vi "HVOF_DAQ.vi"() -> ()   [LabVIEW 2018]
uses:
  <vilib>/Enthought/Python Integration Toolkit/api/Console Visibility.ctl
  Global Variables.vi
  <vilib>/Enthought/Python Integration Toolkit/api/Unpack Double Array.vi
  <resource>/objmgr/daqmx.rc
  <vilib>/Enthought/Python Integration Toolkit/Python Integration Toolkit.lvlib
panel:
  out "Delta T (water)":cluster{"X":dbl[], "Y":dbl[]}(graph)
  in  "Clear Graph":bool=TRUE
  out "XY Graph":cluster{"Y":dbl[], "Y":dbl[]}[](graph)
  in  "Enum":T1(ring)
  out "Data":T2 {"O2 Flow" scale=0.0..600.0; "Fuel Flow" scale=0.0..16.0}
  in  "Temperatures Task Name":refnum<k21>
  in  "Currents Task Name":refnum<k21>
  in  "stop":bool
  # "HVOF"
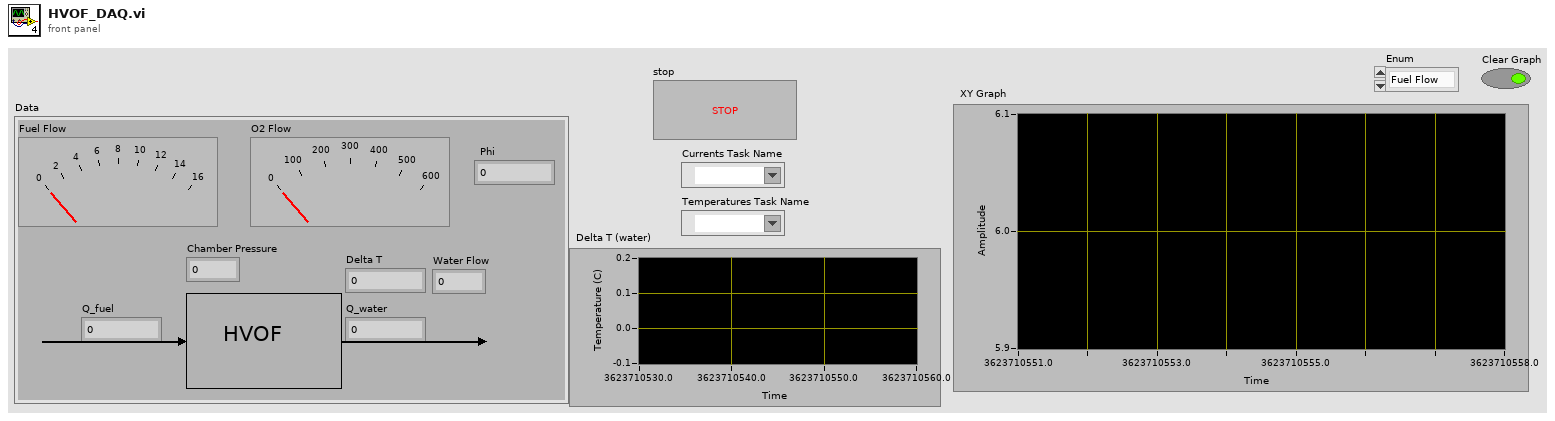
[diagram p1: front panel]
types:
  T1 = enum16{"Fuel Flow", "O2 Flow", "Phi", "Q_water", "Q_Fuel", "Delta T", "Water Flow", "Chamber Pressure"}
  T2 = cluster{"Fuel Flow":dbl, "O2 Flow":dbl, "Phi":dbl, "Q_water":dbl, "Q_fuel":dbl, "Delta T":dbl, "Water Flow":dbl, "Chamber Pressure":dbl}
  T3 = typedef "Python Integration Toolkit.lvlib/Console Visibility.ctl" = enum16{"Show Console", "Show Console While Running", "Hide Console"}
  T4 = typedef "Python Integration Toolkit.lvlib/Session ID.ctl" = u64
  T5 = typedef "Python Integration Toolkit.lvlib/Python Objects.ctl" = variant
  T6 = cluster{dbl, dbl, "Numeric":dbl, "Numeric":dbl, "Numeric":dbl, dbl, dbl, dbl}
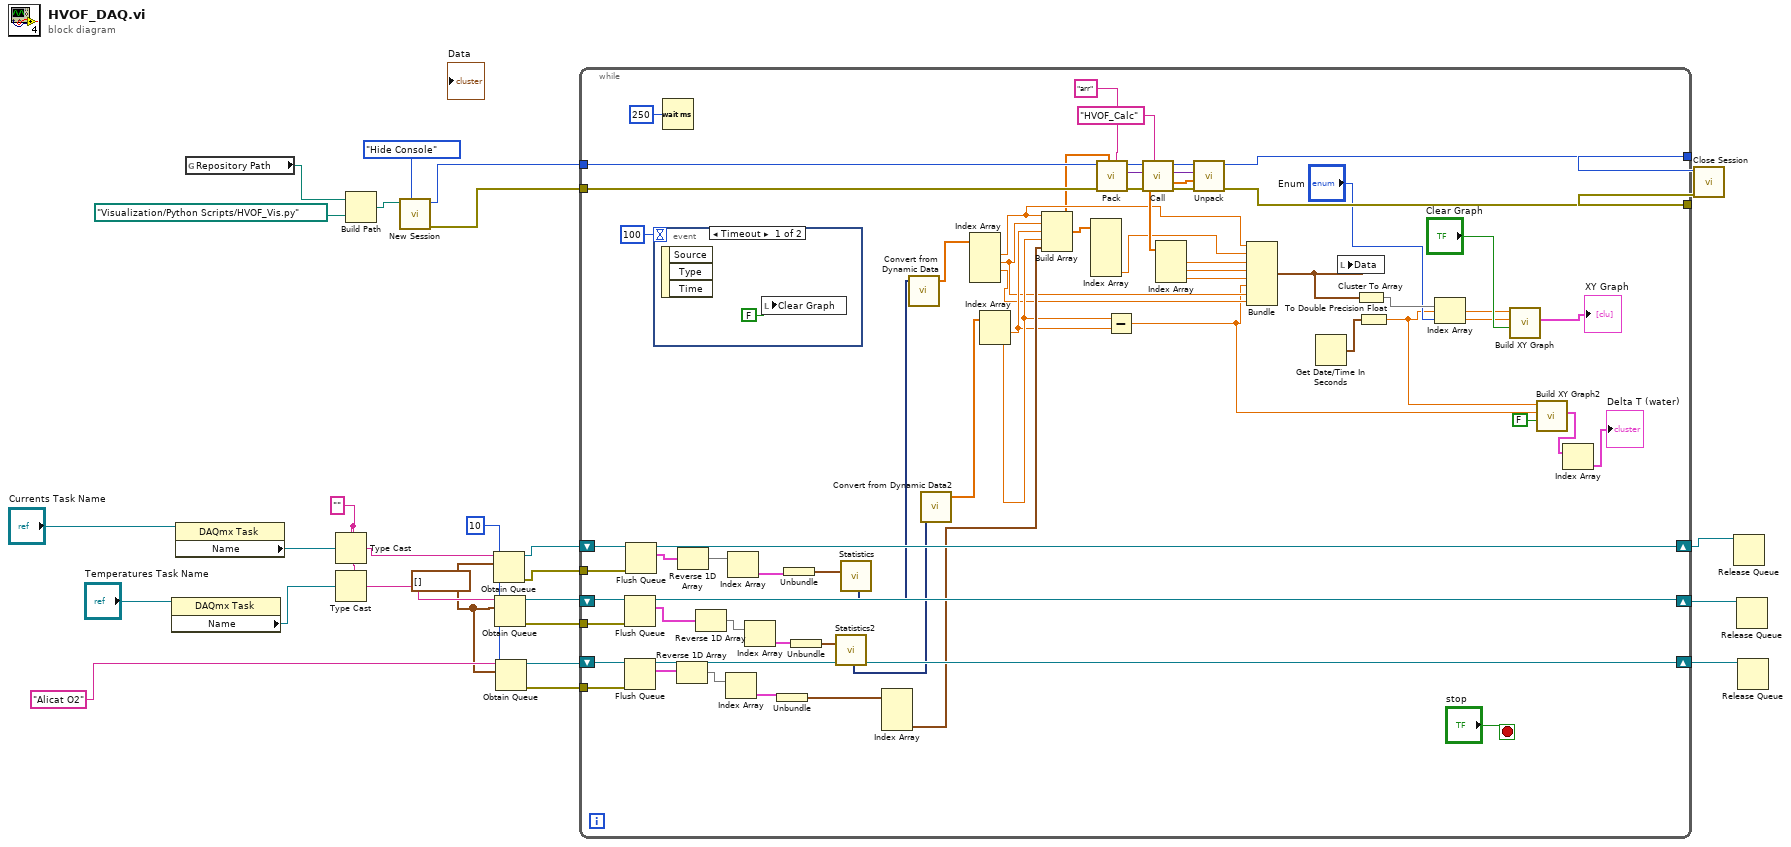
[diagram p0: block diagram]
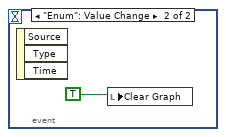
[diagram p2: hidden frame]
diagram:
  w15 = waveform(dbl)[] [] ("data")
  w4 = 10 ("max queue size (-1, unlimited)")
  w25 = "" ("type")
  n1 = property class="DAQmx Task"(reference="Temperatures Task Name") -> ("Name"=w23:refnum<k21>)  [unwired: 1 in, 2 out]
  n2 = property class="DAQmx Task"(reference="Currents Task Name") -> ("Name"=w27:refnum<k21>)  [unwired: 1 in, 2 out]
  n3 = global read "Global Variables.vi" "Repository Path"() -> (w9:path)
  n4 = Type Cast(type=w25, x=w27) -> (*(type *) &x=w26:string)
  n5 = Type Cast(type=w25, x=w23) -> (*(type *) &x=w24:string)
  n6 = Build Path(base path=w9, name or relative path=path "Visualization/Python Scripts/HVOF_Vis.py" ("vi path")) -> (appended path=w11:path)
  n7 = call <vilib>:"New Session.vi"("Console Visibility"=Console_Visibility."Hide Console", "Path to Python Module (.py File)"=w11) -> ("error out"=w7:errorcluster, "Session ID out"=w8:T4)  [unwired: 8 in]
  n8 = Obtain Queue(max queue size (-1, unlimited)=w4, name (unnamed)=w26, element data type=w15) -> (queue out=w20:refnum<queue>, error out=w18:errorcluster)  [unwired: 2 in, 1 out]
  n9 = Obtain Queue(max queue size (-1, unlimited)=w4, name (unnamed)=w24, element data type=w15) -> (queue out=w19:refnum<queue>, error out=w17:errorcluster)  [unwired: 2 in, 1 out]
  n10 = Obtain Queue(max queue size (-1, unlimited)=w4, name (unnamed)="Alicat O2", element data type=w15) -> (queue out=w14:refnum<queue>, error out=w13:errorcluster)  [unwired: 2 in, 1 out]
  n11 = while {
    shift-right: [w87] -> w2
    shift-left: w19 -> [w89]
    shift-right: [w88] -> w3
    shift-left: w20 -> [w90]
    tunnel: w18 -> [w84]
    tunnel: w17 -> [w83]
    shift-right: [w72] -> w1
    shift-left: w14 -> [w75]
    tunnel: w13 -> [w71]
    tunnel: w8 -> [w70]
    tunnel: w7 -> [w69]
    tunnel: [w60] -> w6
    tunnel: [w59] -> w5
    stop <- "stop" stop-if-true
    n12 = Flush Queue(queue=w89, error in (no error)=w83) -> (queue out=w87:refnum<queue>, remaining elements=w86:cluster{"data":waveform(dbl)[]}[])  [unwired: 1 out]
    n13 = Flush Queue(queue=w75, error in (no error)=w71) -> (queue out=w72:refnum<queue>, remaining elements=w73:cluster{"data":waveform(dbl)[]}[])  [unwired: 1 out]
    n14 = Flush Queue(queue=w90, error in (no error)=w84) -> (queue out=w88:refnum<queue>, remaining elements=w85:cluster{"data":waveform(dbl)[]}[])  [unwired: 1 out]
    n15 = event shown="[0] Timeout" {
      selector: _ -> [_ _]
      dyn-events: _ -> [_ _]
      timeout: 100 -> [_ _]
      event Timeout {
        n16 = event-data() -> ()  [unwired: 1 in, 3 out]
        n17 = local write "Clear Graph"(FALSE) -> ()
      }
      event "Enum": Value Change {
        n18 = event-data() -> ()  [unwired: 1 in, 3 out]
        n19 = local write "Clear Graph"(TRUE) -> ()
      }
    }
    n20 = Wait (ms)(milliseconds to wait=u32 250) -> ()  [unwired: 1 out]
    n21 = Reverse 1D Array(array=w73) -> (reversed array=w74:cluster{"data":waveform(dbl)[]}[])
    n22 = Reverse 1D Array(array=w85) -> (reversed array=w82:cluster{"data":waveform(dbl)[]}[])
    n23 = Reverse 1D Array(array=w86) -> (reversed array=w81:cluster{"data":waveform(dbl)[]}[])
    n24 = Index Array(array=w74) -> (element=w54:cluster{"data":waveform(dbl)[]})  [unwired: 1 in]
    n25 = Index Array(array=w82) -> (element=w80:cluster{"data":waveform(dbl)[]})  [unwired: 1 in]
    n26 = Index Array(array=w81) -> (element=w79:cluster{"data":waveform(dbl)[]})  [unwired: 1 in]
    n27 = Unbundle(w54) -> ("data"=w53:waveform(dbl)[])
    n28 = Unbundle(w80) -> ("data"=w77:waveform(dbl)[])
    n29 = Unbundle(w79) -> ("data"=w76:waveform(dbl)[])
    n30 = call "Statistics2"("Signals"=w76) -> ("Arithmetic Mean"=w57:dynamicdata)  [unwired: 25 in, 1 out]
    n31 = call "Statistics"("Signals"=w77) -> ("Arithmetic Mean"=w58:dynamicdata)  [unwired: 25 in, 1 out]
    n32 = Index Array(array=w53) -> (element #3=w47:waveform(dbl))  [unwired: 3 in, 2 out]
    n33 = call "Convert from Dynamic Data"("Dynamic Data Type"=w58) -> ("Array"=w56:dbl[])  [unwired: 3 in]
    n34 = call "Convert from Dynamic Data2"("Dynamic Data Type"=w57) -> ("Array"=w55:dbl[])  [unwired: 3 in]
    n35 = Index Array(array=w56) -> (element #1=w48:dbl, element #2=w35:dbl, element #3=w34:dbl)  [unwired: 4 in, 1 out]
    n36 = Index Array(array=w55) -> (element #1=w45:dbl, element #2=w46:dbl)  [unwired: 2 in]
    n37 = Build Array(w48, w35, w45, w46, w47) -> (w43:dbl[])
    n38 = Index Array(array=w43) -> (element #5=w42:dbl)  [unwired: 5 in, 4 out]
    n39 = call <vilib>:"Pack.vi"("Keyword Name"="arr", "Argument"=w43, "error in (no error)"=w69, "Session ID"=w70) -> ("error out"=w68:errorcluster, "Python Object References Out"=w67:T5, "Session ID out"=w66:T4)  [unwired: 5 in]
    n40 = Subtract(x=w46, y=w45) -> (x-y=w33:dbl)
    n41 = call <vilib>:"Call.vi"("Function or Method Name"="HVOF_Calc" ("Python Code"), "error in (no error)"=w68, "Python Object References In"=w67, "Session ID"=w66) -> ("error out"=w63:errorcluster, "Python Object References Out"=w62:T5, "Session ID out"=w61:T4)  [unwired: 5 in]
    n42 = call-poly <vilib>:"Unpack.vi"("error in (no error)"=w63, "Python Object References In"=w62, "Session ID"=w61) -> ("error out"=w59:errorcluster, "Value"=w52:dbl[], "Session ID out"=w60:T4)  [unwired: 5 in, 1 out]
    n43 = Index Array(array=w52) -> (element #1=w51:dbl, element #2=w50:dbl, element #3=w49:dbl)  [unwired: 3 in]
    n44 = Bundle(w48, w42, "Numeric"=w51, "Numeric"=w50, "Numeric"=w49, w33, w35, w34) -> (w44:T6)  [unwired: 1 in]
    n45 = Get Date/Time In Seconds() -> (seconds since 1Jan1904=w30:timestamp)
    n46 = local write "Data"(w44) -> ()
    n47 = Cluster To Array(cluster=w44) -> (array=w39:dbl[])
    n48 = To Double Precision Float(number=w30) -> (double precision float=w32:dbl)
    n49 = Index Array(array=w39, index="Enum") -> (element=w37:dbl)
    n50 = call "Build XY Graph"("Reset"="Clear Graph", "Y Input"=w37, "X Input"=w32) -> ("XY Graph"=→"XY Graph":cluster{"X":dbl[], "Y":dbl[]}[])  [unwired: 7 in, 1 out]
    n51 = call "Build XY Graph2"("Reset"=FALSE, "Y Input"=w33, "X Input"=w32) -> ("XY Graph"=w28:cluster{"X":dbl[], "Y":dbl[]}[])  [unwired: 7 in, 1 out]
    n52 = Index Array(array=w28) -> (element=→"Delta T (water)":cluster{"X":dbl[], "Y":dbl[]})  [unwired: 1 in]
  }
  n53 = call <vilib>:"Close Session.vi"("error in (no error)"=w5, "Session ID"=w6) -> ()  [unwired: 9 in, 1 out]
  n54 = Release Queue(queue=w3) -> ()  [unwired: 2 in, 3 out]
  n55 = Release Queue(queue=w2) -> ()  [unwired: 2 in, 3 out]
  n56 = Release Queue(queue=w1) -> ()  [unwired: 2 in, 3 out]
